vi "YTO_Zero_Corr_Voltage_Naoj.vi"(0 "ObjHandle in":u32, 2 "Desired YTO Corr Volt [V]":dbl, 3 "Voltage Limit [mV]":dbl, 5 "error in (no error)":errorcluster, 8 "Slave Node in":cluster{"Address":i16, "Serial Number":i8[]}={"Address"=19, "Serial Number"=[16, 71, 55, 76, 1, 8, 0, -15]} {"Serial Number" format="%.0x"; "Address" format="%.0x"}, 9 "SET YTO COARSE TUNE":sgl min=0 max=42 step=1 format="%.2f", 11 "YTO Low freq. [GHz]":sgl=12.17 format="%.3f", 12 "Cartridge band":u32 max=10 step=1, 13 "YTO High freq. [GHz]":sgl=14.833 format="%.3f") -> (14 "ObjHandle out":u32, 16 "YTO_fine":dbl, 17 "corrV":dbl, 19 "error out":errorcluster)   [LabVIEW 2017]
panel:
  in  "step(GHz)":sgl=0.001
  # "Node Address"
  # "Serial Number"
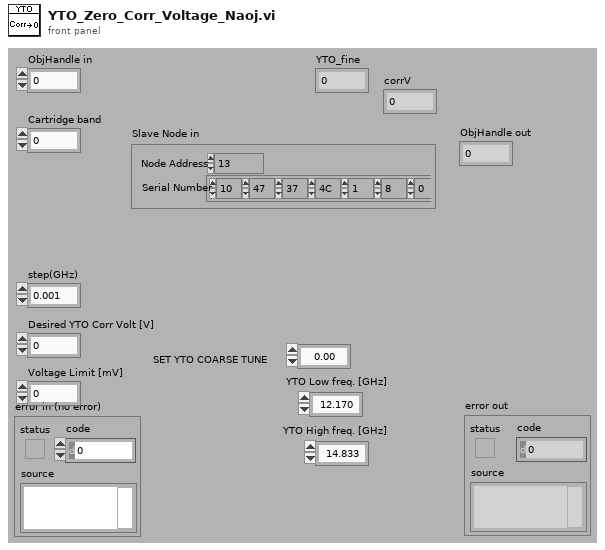
[diagram p1: front panel]
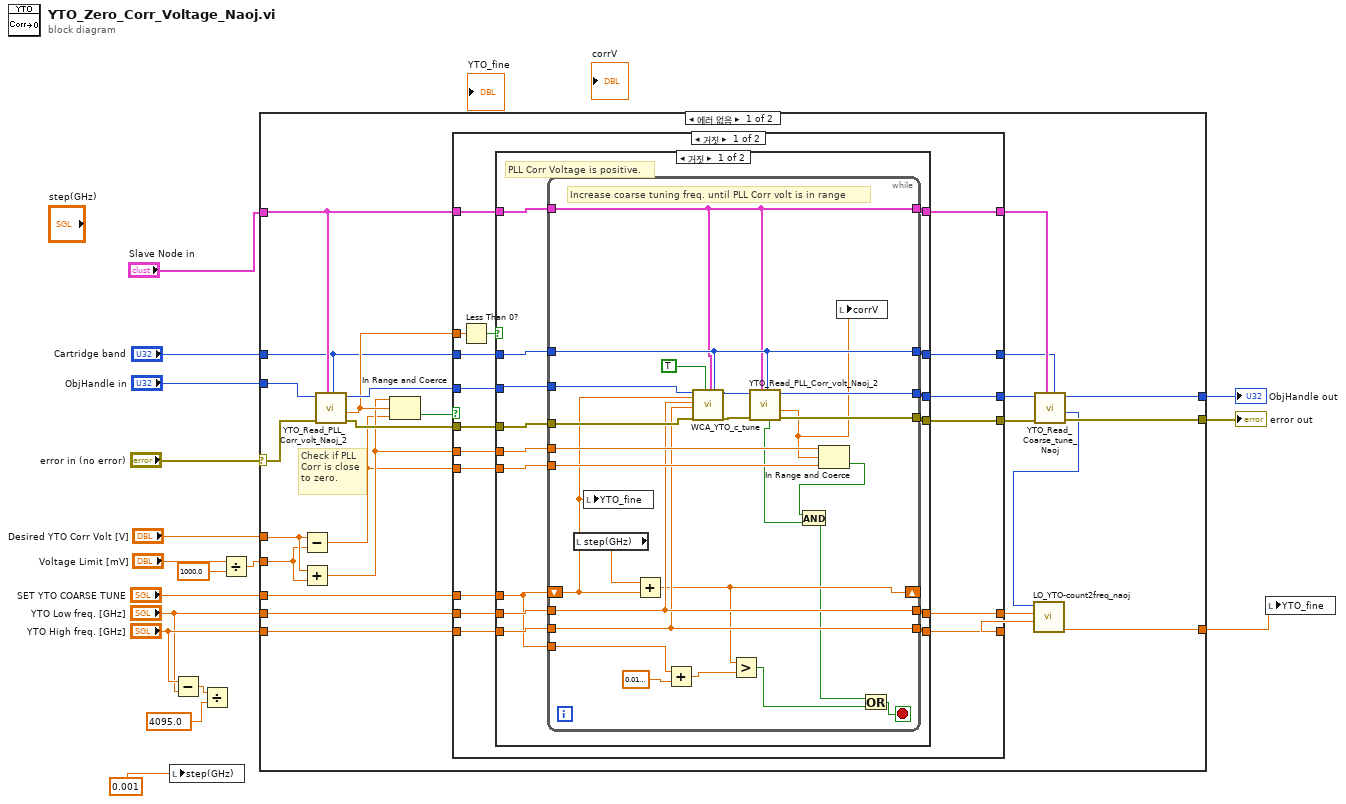
[diagram p0: block diagram]
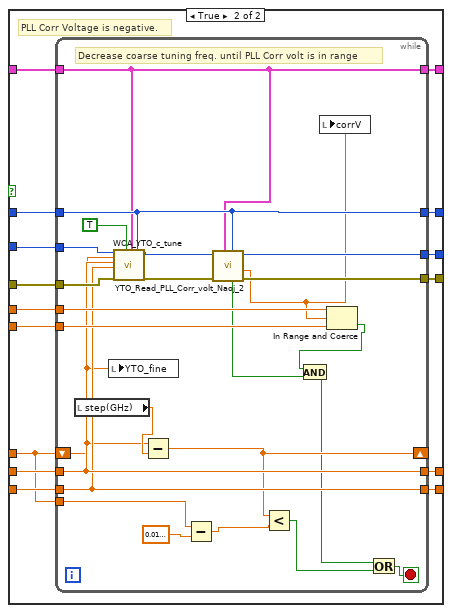
[diagram p2: hidden frame]
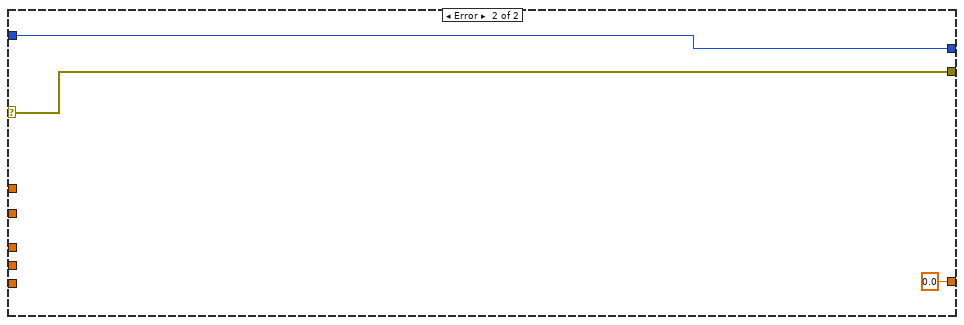
[diagram p4: hidden frame]
diagram:
  n1 = local write "step(GHz)"(0.001) -> ()
  n2 = Subtract(x="YTO High freq. [GHz]", y="YTO Low freq. [GHz]") -> (x-y=w4:sgl)
  n3 = Divide(x=w4, y=4095.0) -> ()  [unwired: 1 out]
  n4 = Divide(x="Voltage Limit [mV]", y=1000.0) -> (x/y=w10:dbl)
  n5 = case shown="에러 없음" "error in (no error)" {
    selector: "error in (no error)" -> [w41 w147]
    tunnel: "ObjHandle in" -> [w42 w148]
    tunnel: "Slave Node in" -> [w31 _]
    tunnel: "Desired YTO Corr Volt [V]" -> [w40 _]
    tunnel: w10 -> [w39 _]
    tunnel: [w26 w148] -> w14
    tunnel: [w25 w147] -> w13
    tunnel: "SET YTO COARSE TUNE" -> [w34 _]
    tunnel: "YTO Low freq. [GHz]" -> [w33 _]
    tunnel: "YTO High freq. [GHz]" -> [w32 _]
    tunnel: [w20 sgl 0.0 ("YTO freq.")] -> w1
    tunnel: "Cartridge band" -> [w19 _]
    frame No Error {
      # "Check if PLL\nCorr is close\nto zero."
      n6 = Subtract(x=w40, y=w39) -> (x-y=w29:dbl)
      n7 = Add(x=w40, y=w39) -> (x+y=w30:dbl)
      n8 = call "YTO_Read_PLL_Corr_volt_Naoj_2.vi"("Cartridge band"=w19, "Slave Node in"=w31, "error IO"=w41, "ObjHandle in"=w42) -> ("error"=w36:errorcluster, "PLL Corr Voltage [V]"=w35:sgl, "ObjHandle out"=w37:u32)  [unwired: 4 in, 1 out]
      n9 = In Range and Coerce(upper limit=w30, x=w35, lower limit=w29) -> (In Range?=w38:bool)  [unwired: 1 out]
      n10 = case shown="거짓" w38 {
        tunnel: w37 -> [w57 w145]
        tunnel: w36 -> [w56 w144]
        tunnel: [w49 w145] -> w28
        tunnel: [w48 w144] -> w27
        tunnel: w35 -> [w59 _]
        tunnel: w34 -> [w55 _]
        tunnel: w33 -> [w54 w142]
        tunnel: w32 -> [w53 w141]
        tunnel: w31 -> [w52 w143]
        tunnel: w30 -> [w51 _]
        tunnel: w29 -> [w50 _]
        tunnel: [w47 w143] -> w24
        tunnel: [w46 w142] -> w23
        tunnel: [w45 w141] -> w22
        tunnel: w19 -> [w44 w140]
        tunnel: [w43 w140] -> w18
        frame False {
          n11 = Less Than 0?(x=w59) -> (x < 0?=w58:bool)
          n12 = case shown="거짓" w58 {
            tunnel: w57 -> [w74 w114]
            tunnel: w56 -> [w73 w113]
            tunnel: w55 -> [w60 w100]
            tunnel: w54 -> [w72 w112]
            tunnel: w53 -> [w71 w111]
            tunnel: w52 -> [w70 w110]
            tunnel: w51 -> [w69 w109]
            tunnel: w50 -> [w68 w108]
            tunnel: [w67 w107] -> w49
            tunnel: [w66 w106] -> w48
            tunnel: [w65 w105] -> w47
            tunnel: [w64 w104] -> w46
            tunnel: [w63 w103] -> w45
            tunnel: w44 -> [w62 w102]
            tunnel: [w61 w101] -> w43
            frame False {
              # "PLL Corr Voltage is positive."
              n13 = while {
                tunnel: w74 -> [w99]
                tunnel: w73 -> [w98]
                tunnel: w72 -> [w88]
                tunnel: w71 -> [w87]
                tunnel: w70 -> [w86]
                tunnel: w69 -> [w94]
                tunnel: w68 -> [w93]
                tunnel: [w92] -> w67
                tunnel: [w91] -> w66
                shift-right: [w82] -> _
                shift-left: w60 -> [w79]
                tunnel: [w86] -> w65
                tunnel: [w88] -> w64
                tunnel: [w87] -> w63
                tunnel: w62 -> [w90]
                tunnel: [w90] -> w61
                tunnel: w60 -> [w84]
                stop <- w89 stop-if-true
                # "Increase coarse tuning freq. until PLL Corr volt is in range"
                n14 = local read "step(GHz)"() -> (w80:sgl)
                n15 = local write "YTO_fine"(w79) -> ()
                n16 = Add(x=w80, y=w79) -> (x+y=w82:sgl)
                n17 = Add(x=w84, y=sgl 0.02 ("x")) -> (x+y=w83:sgl)
                n18 = call "WCA_YTO_c_tune.vi"("ObjHandle in"=w99, "SET YTO COARSE TUNE"=w79, "YTO Low freq. [GHz]"=w88, "YTO High freq. [GHz]"=w87, "error in (no error)"=w98, "LO locked?"=TRUE, "Slave Node in"=w86, "Cartridge band"=w90) -> ("ObjHandle out"=w96:u32, "error out"=w95:errorcluster)  [unwired: 10 in]
                n19 = Greater?(x=w82, y=w83) -> (0:w81:bool)
                n20 = call "YTO_Read_PLL_Corr_volt_Naoj_2.vi"("Cartridge band"=w90, "Slave Node in"=w86, "error IO"=w95, "ObjHandle in"=w96) -> ("error"=w91:errorcluster, "PLL Corr Voltage [V]"=w78:sgl, "ObjHandle out"=w92:u32, "Lock??"=w77:bool)  [unwired: 4 in]
                n21 = In Range and Coerce(upper limit=w94, x=w78, lower limit=w93) -> (In Range?=w75:bool)  [unwired: 1 out]
                n22 = And(x=w75, y=w77) -> (x .and. y?=w76:bool)
                n23 = local write "corrV"(w78) -> ()
                n24 = Or(x=w76, y=w81) -> (x .or. y?=w89:bool)
              }
            }
            frame True {
              # "PLL Corr Voltage is negative."
              n25 = while {
                tunnel: w114 -> [w139]
                tunnel: w113 -> [w138]
                tunnel: w112 -> [w129]
                tunnel: w111 -> [w128]
                tunnel: w110 -> [w126]
                tunnel: w109 -> [w134]
                tunnel: w108 -> [w133]
                tunnel: [w132] -> w107
                tunnel: [w131] -> w106
                shift-right: [w122] -> _
                shift-left: w100 -> [w119]
                tunnel: [w126] -> w105
                tunnel: [w129] -> w104
                tunnel: [w128] -> w103
                tunnel: w102 -> [w130]
                tunnel: [w130] -> w101
                tunnel: w100 -> [w124]
                stop <- w127 stop-if-true
                # "Decrease coarse tuning freq. until PLL Corr volt is in range"
                n26 = local read "step(GHz)"() -> (w120:sgl)
                n27 = local write "YTO_fine"(w119) -> ()
                n28 = call "WCA_YTO_c_tune.vi"("ObjHandle in"=w139, "SET YTO COARSE TUNE"=w119, "YTO Low freq. [GHz]"=w129, "YTO High freq. [GHz]"=w128, "error in (no error)"=w138, "LO locked?"=TRUE, "Slave Node in"=w126, "Cartridge band"=w130) -> ("ObjHandle out"=w136:u32, "error out"=w135:errorcluster)  [unwired: 10 in]
                n29 = Subtract(x=w119, y=w120) -> (x-y=w122:sgl)
                n30 = Subtract(x=w124, y=sgl 0.02 ("x")) -> (x-y=w123:sgl)
                n31 = call "YTO_Read_PLL_Corr_volt_Naoj_2.vi"("Cartridge band"=w130, "Slave Node in"=w126, "error IO"=w135, "ObjHandle in"=w136) -> ("error"=w131:errorcluster, "PLL Corr Voltage [V]"=w118:sgl, "ObjHandle out"=w132:u32, "Lock??"=w117:bool)  [unwired: 4 in]
                n32 = Less?(x=w122, y=w123) -> (x < y?=w121:bool)
                n33 = local write "corrV"(w118) -> ()
                n34 = In Range and Coerce(upper limit=w134, x=w118, lower limit=w133) -> (In Range?=w116:bool)  [unwired: 1 out]
                n35 = And(x=w116, y=w117) -> (x .and. y?=w115:bool)
                n36 = Or(x=w115, y=w121) -> (x .or. y?=w127:bool)
              }
            }
          }
        }
        frame True {
          # "No coarse tuning neded."
        }
      }
      n37 = call "YTO_Read_Coarse_tune_Naoj.vi"("Cartridge band"=w18, "Slave Node in"=w24, "error IO"=w27, "ObjHandle in"=w28) -> ("error"=w25:errorcluster, "YTO Coarse Tune"=w21:u16, "ObjHandle out"=w26:u32)  [unwired: 5 in]
      n38 = call "LO_YTO-count2freq_naoj.vi"("f max"=w22, "f min"=w23, "YTO count"=w21) -> ("YTO freq."=w20:sgl)  [unwired: 6 in]
    }
    frame Error {
    }
  }
  "error out" <- w13
  "ObjHandle out" <- w14
  n39 = local write "YTO_fine"(w1) -> ()
